vi "experiment control.vi"() -> ()   [LabVIEW 2012] (continued)
                    n363 = Greater Or Equal?(x=w828, y=w827) -> (x >= y?=w826:bool)
                    n364 = Greater?(x=w827, y=w829) -> (0:w825:bool)
                    n365 = And(x=w826, y=w825) -> (x .and. y?=w823:bool)
                  }
                  frame "TiSapph" {
                    n366 = local read "TiSapph"() -> (w833:T18)
                    n367 = Unbundle By Name(w833) -> ("scan start"=w840:dbl, "setpoint"=w836:dbl, "scan end"=w839:dbl)
                    n368 = Max & Min(x=w840, y=w839) -> (max(x,y)=w837:dbl, min(x,y)=w838:dbl)
                    n369 = Greater Or Equal?(x=w837, y=w836) -> (x >= y?=w835:bool)
                    n370 = Greater?(x=w836, y=w838) -> (0:w834:bool)
                    n371 = And(x=w835, y=w834) -> (x .and. y?=w832:bool)
                  }
                  frame "Scan" {
                    n372 = case shown="\"\"" w841 {
                      tunnel: [w849 w850] -> w842
                      tunnel: w841 -> [w843 _]
                      frame Default {
                        n373 = local read "Scan References"() -> (w848:T33)
                        n374 = Decimal String To Number(string=w843) -> (number=w847:i32)  [unwired: 2 in, 1 out]
                        n375 = Index Array(array=w848, index=w847) -> (element=w846:T57)
                        n376 = Unbundle By Name(w846) -> ("progress"=w845:u8)
                        n377 = Less?(x=w845, y=u8 100) -> (x < y?=w849:bool)
                      }
                      frame "" {
                        n378 = local read "Scan References"() -> (w852:T33)
                        n379 = for {
                          tunnel: w852 -> [w858] mode=indexing
                          tunnel: [w854] -> w851 mode=indexing
                          n380 = Unbundle By Name(w858) -> ("scan"=w853:bool, "progress"=w857:u8)
                          n381 = Less?(x=w857, y=u8 100) -> (x < y?=w855:bool)
                          n382 = And(x=w853, y=w855) -> (x .and. y?=w854:bool)
                        }
                        n383 = Or Array Elements(Boolean array=w851) -> (logical OR=w850:bool)
                      }
                    }
                  }
                  frame "Switch" {
                    n384 = local read "Slide"() -> (w859:u8)
                    n385 = Less?(x=w859, y=u8 100) -> (x < y?=w861:bool)
                  }
                }
                n386 = case shown="True" w783 {
                  tunnel: w781 -> [_ w794]
                  tunnel: w785 -> [_ w793]
                  tunnel: [w791 w792] -> w784
                  tunnel: w782 -> [w791 _]
                  frame False {
                  }
                  frame True {
                    n387 = Build Array (concatenate)(w793, w794) -> (w792:string[])
                  }
                }
              }
            }
            n388 = Reverse 1D Array(array=w765) -> (reversed array=w768:string[])
            n389 = for {
              tunnel: w769 -> [w777]
              tunnel: w768 -> [w774] mode=indexing
              shift-right: [w775] -> w766
              shift-left: w767 -> [w776]
              n390 = Enqueue Element At Opposite End(queue=w777, element=w774, error in (no error)=w776) -> (error out=w775:errorcluster)  [unwired: 1 in, 2 out]
            }
          }
          frame "Count Ions" {
            # "This command calls the custom functions specified in the programming tab"
            n391 = Index Array(array=w883) -> (element=w882:string)  [unwired: 1 in]
            n392 = Unbundle By Name(w919) -> ("TDS5034B Data"=w915:cluster{"Y":dbl[], "t0":dbl, "dt":dbl}[])
            n393 = Decimal String To Number(string=w882) -> (number=w916:i32)  [unwired: 2 in, 1 out]
            n394 = Unbundle By Name("Count Ions") -> ("Hf  time threshold"=w900:dbl, "Ion Calibration"=w901:dbl, "Hf integrated history"=w898:dbl[], "HfF history"=w897:dbl[], "History"=w886:u32, "Clear History"=w887:bool)
            n395 = Index Array(array=w915, index=w916) -> (element=w917:cluster{"Y":dbl[], "t0":dbl, "dt":dbl})
            n396 = Unbundle By Name(w917) -> ("Y"=w910:dbl[], "dt"=w902:dbl)
            n397 = Select(t=u32 1, s=w887, f=w886) -> (s? t:f=w885:u32)
            n398 = Array Subset(array=w910, length=500) -> (w913:dbl[])  [unwired: 1 in]
            n399 = call-poly <vilib>:"Mean.vi"("X"=w913) -> ("mean"=w911:dbl)  [unwired: 1 out]
            n400 = Subtract(x=w910, y=w911) -> (x-y=w909:dbl[])
            n401 = Divide(x=w900, y=w902) -> (x/y=w912:dbl)
            n402 = Split 1D Array(array=w909, index=w912) -> (first subarray=w908:dbl[], second subarray=w907:dbl[])
            n403 = Add Array Elements(numeric array=w908) -> (sum=w903:dbl)
            n404 = Add Array Elements(numeric array=w907) -> (sum=w904:dbl)
            n405 = Multiply(x=w902, y=w903) -> (x*y=w906:dbl)
            n406 = Multiply(x=w902, y=w904) -> (x*y=w905:dbl)
            n407 = Divide(x=w906, y=w901) -> (x/y=w896:dbl)
            n408 = Divide(x=w905, y=w901) -> (x/y=w895:dbl)
            n409 = Build Array (concatenate)(w896, w898) -> (w893:dbl[])
            n410 = Build Array (concatenate)(w895, w897) -> (w892:dbl[])
            n411 = Array Subset(array=w893, length=w885) -> (w889:dbl[])  [unwired: 1 in]
            n412 = Array Subset(array=w892, length=w885) -> (w888:dbl[])  [unwired: 1 in]
            n413 = call-poly <vilib>:"Mean.vi"("X"=w889) -> ("mean"=w890:dbl)  [unwired: 1 out]
            n414 = call-poly <vilib>:"Mean.vi"("X"=w888) -> ("mean"=w891:dbl)  [unwired: 1 out]
            n415 = Bundle By Name(cluster="Count Ions", "Hf integrated"=w896, "HfF"=w895, "Hf integrated history"=w889, "HfF history"=w888, "<Hf integrated>"=w890, "<HfF>"=w891) -> (w894:T34)
            n416 = local write "Count Ions"(w894) -> ()
          }
          frame "uBinary: Save" {
            # "Saves a uBinary file or loads a uBinary file."
            n417 = flat-sequence {
              tunnel: [w933] -> w923
              tunnel: w927 -> [w933]
              tunnel: w921 -> [w928]
              frame #0 {
                n418 = Unbundle By Name(w928) -> ("TDS5034B Data"=→"TDS5034B Data":cluster{"Y":dbl[], "t0":dbl, "dt":dbl}[])
                n419 = Get Date/Time String(want seconds? (F)=TRUE) -> (date string=w931:string, time string=w932:string)  [unwired: 2 in]
                n420 = local write "Time"(w932) -> ()
                n421 = local write "Date"(w931) -> ()
              }
            }
            n422 = case shown="\"Scan\"" w925 {
              selector: w925 -> [_ _ w1085 _]
              tunnel: w923 -> [w940 w960 w1086 w1092]
              tunnel: [w936 w963 w1089 w1091] -> w926
              tunnel: [w934 w962 w1088 w1096] -> w924
              tunnel: w921 -> [w934 w962 w1088 w1097]
              frame "Prompt" {
                n423 = Format Date/Time String(time format string (%c)="%Y") -> (date/time string=w943:string)  [unwired: 2 in]
                n424 = Format Date/Time String(time format string (%c)="\\%y%m%d\\") -> (date/time string=w941:string)  [unwired: 2 in]
                n425 = Concatenate Strings("X:\\" ("string"), w943, w941) -> (w946:string)
                n426 = String To Path(string=w946) -> (path=w949:path)
                n427 = call "File Dialog3"("start path"=w949, "prompt"="Save Experiment (*.ubin)", "button label"="Save", "error in"=w940, "pattern (all files)"="*.ubin") -> ("selected path"=w938:path, "error out"=w939:errorcluster)  [unwired: 7 in, 2 out]
                n428 = control-ref of="This VI"() -> (w937:refnum<vi>)
                n429 = call "ubinary_save.vi"("error in"=w939, "file (use dialog)"=w938, "VI"=w937) -> ("error out"=w936:errorcluster)  [unwired: 8 in]
              }
              frame "" {
                n430 = local read "Working Directory"() -> (w952:path)
                n431 = List Folder(path=w952, error in=w960) -> (filenames=w951:string[], error out=w959:errorcluster)  [unwired: 2 in, 2 out]
                n432 = Path To String(path=w952) -> (string=w954:string)
                n433 = Array Size(array=w951) -> (size(s)=w950:i32)
                n434 = case shown="Default" w950 {
                  tunnel: w951 -> [_ w969]
                  tunnel: [1 w966] -> w958
                  frame 0 {
                  }
                  frame Default {
                    n435 = for {
                      tunnel: w969 -> [w973] mode=indexing
                      tunnel: [w971] -> w968 mode=indexing
                      n436 = xnode "Match Regular Expression"("input string"=w973, "regular expression"="\\d+") -> ("whole match"=w972:string)  [unwired: 4 in, 4 out]
                      n437 = Decimal String To Number(string=w972) -> (number=w971:i32)  [unwired: 2 in, 1 out]
                    }
                    n438 = Array Max & Min(array=w968) -> (max value=w967:i32)  [unwired: 3 out]
                    n439 = Increment(x=w967) -> (x+1=w966:i32)
                  }
                }
                n440 = Number To Decimal String(number=w958) -> (decimal integer string=w957:string)  [unwired: 1 in]
                n441 = Concatenate Strings(w954, "\\s" ("string"), w957, ".ubin" ("string")) -> (w955:string)
                n442 = control-ref of="This VI"() -> (w964:refnum<vi>)
                n443 = String To Path(string=w955) -> (path=w961:path)
                n444 = call "ubinary_save.vi"("error in"=w959, "file (use dialog)"=w961, "VI"=w964) -> ("error out"=w963:errorcluster)  [unwired: 8 in]
              }
              frame Default {
                n445 = control-ref of="This VI"() -> (w1090:refnum<vi>)
                n446 = String To Path(string=w1085) -> (path=w1087:path)
                n447 = call "ubinary_save.vi"("error in"=w1086, "file (use dialog)"=w1087, "VI"=w1090) -> ("error out"=w1089:errorcluster)  [unwired: 8 in]
              }
              frame "Scan" {
                w1105 = "." ("substring (\"\")")
                n448 = Unbundle By Name(w1097) -> ("Scan Index"=w1098:u32, "Scan Prefix"=w1099:path, "Scan Index"=w1095:u32)
                n449 = Number To Decimal String(number=w1095) -> (decimal integer string=w1103:string)  [unwired: 1 in]
                n450 = Strip Path(path=w1099) -> (stripped path=w1101:path, name=w1106:string)
                n451 = Concatenate Strings(w1103, w1105) -> (w1104:string)
                n452 = Increment(x=w1098) -> (x+1=w1100:u32)
                n453 = Search and Replace String(input string=w1106, search string=w1105, replace string=w1104) -> (result string=w1102:string)  [unwired: 5 in, 3 out]
                n454 = Bundle By Name(cluster=w1097, "Scan Index"=w1100) -> (w1096:T52)
                n455 = Build Path(base path=w1101, name or relative path=w1102) -> (appended path=w1093:path)
                n456 = control-ref of="This VI"() -> (w1094:refnum<vi>)
                n457 = call "ubinary_save.vi"("error in"=w1092, "file (use dialog)"=w1093, "VI"=w1094) -> ("error out"=w1091:errorcluster)  [unwired: 8 in]
              }
            }
          }
          frame "uBinary: Load" {
            # "Saves a uBinary file or loads a uBinary file."
            n458 = Index Array(array=w1108, index=0) -> (element=w1107:string)
            n459 = Index Array(array=w1108, index=1) -> (element=w1111:string)
            n460 = case shown="\"False\", Default" w1111 {
              selector: w1111 -> [w1119 _]
              tunnel: w1115 -> [w1121 w1134]
              tunnel: [w1121 w1124] -> w1114
              tunnel: [w1120 w1123] -> w1113
              frame "False", Default {
                n461 = String To Path(string=w1119) -> (path=w1120:path)
              }
              frame "" {
                n462 = Format Date/Time String(time format string (%c)="%Y") -> (date/time string=w1127:string)  [unwired: 2 in]
                n463 = Format Date/Time String(time format string (%c)="\\%y%m%d\\") -> (date/time string=w1125:string)  [unwired: 2 in]
                n464 = Concatenate Strings("X:\\" ("string"), w1127, w1125) -> (w1130:string)
                n465 = String To Path(string=w1130) -> (path=w1133:path)
                n466 = call "File Dialog2"("start path"=w1133, "prompt"="Load Experiment (*.ubin)", "button label"="Load", "error in"=w1134, "pattern (all files)"="*.ubin") -> ("selected path"=w1123:path, "error out"=w1124:errorcluster)  [unwired: 7 in, 2 out]
              }
            }
            n467 = control-ref of="This VI"() -> (w1112:refnum<vi>)
            n468 = call "ubinary_load.vi"("error in"=w1114, "control"=w1107, "file (use dialog)"=w1113, "VI"=w1112) -> ("error out"=w1118:errorcluster)  [unwired: 7 in]
          }
          frame "uBinary2" {
            # "First, modify Save"
            # "Saves a uBinary file or loads a uBinary file."
            n469 = Match Pattern(string=w1144, regular expression=",") -> (before substring=w1138:string, after substring=w1136:string, offset past match=w1137:i32)  [unwired: 1 in, 1 out]
            n470 = case shown="\"Load\"" w1138 {
              tunnel: [w1153 w1400 w1421] -> w1142
              tunnel: w1143 -> [w1145 w1399 w1423]
              tunnel: w1140 -> [w1146 _ w1419]
              tunnel: [w1149 w1402 w1418] -> w1141
              tunnel: w1140 -> [w1149 w1401 w1417]
              tunnel: w1137 -> [w1148 _ _]
              tunnel: w1136 -> [w1147 _ _]
              tunnel: w1135 -> [_ w1394 w1413]
              frame "Save", Default {
                n471 = case shown="0, Default" w1148 {
                  tunnel: w1145 -> [w1156 w1161]
                  tunnel: [w1156 w1160] -> w1152
                  tunnel: [w1154 w1159] -> w1151
                  tunnel: [FALSE ("cancelled") w1158] -> w1150
                  tunnel: w1147 -> [w1155 _]
                  frame 0, Default {
                    n472 = String To Path(string=w1155) -> (path=w1154:path)
                  }
                  frame -1 {
                    n473 = Format Date/Time String(time format string (%c)="%Y") -> (date/time string=w1164:string)  [unwired: 2 in]
                    n474 = Format Date/Time String(time format string (%c)="\\%y%m%d\\") -> (date/time string=w1162:string)  [unwired: 2 in]
                    n475 = Concatenate Strings("X:\\" ("string"), w1164, w1162) -> (w1167:string)
                    n476 = String To Path(string=w1167) -> (path=w1170:path)
                    n477 = call "File Dialog4"("start path"=w1170, "prompt"="Save Experiment (*.ubin)", "button label"="Save", "error in"=w1161) -> ("selected path"=w1159:path, "cancelled"=w1158:bool, "error out"=w1160:errorcluster)  [unwired: 8 in, 1 out]
                  }
                }
                n478 = case shown="False" w1150 {
                  tunnel: [w1174 w1393] -> w1153
                  tunnel: w1152 -> [w1173 w1393]
                  tunnel: w1151 -> [w1172 _]
                  tunnel: w1146 -> [w1171 _]
                  frame False {
                    # "Then add a case to handle the tag"
                    # "Add your tag to the list"
                    n479 = call "begin_ubin.vi"("error in"=w1173, "file"=w1172) -> ("error out"=w1178:errorcluster, "refnum out"=w1179:refnum<file>)  [unwired: 8 in]
                    n480 = for {
                      tunnel: string[] ["Time", "DIO64", "DAC", "Scan", "Lasers", "AOM DDS", "Trap DDS", "Commands", "Wavemaster", "Frequency", "Microwave", "Measurements", "Switches", "Data", "Trap"] -> [w1181] mode=indexing
                      shift-right: [w1183] -> w1177
                      shift-left: w1179 -> [w1185]
                      shift-right: [w1182] -> w1176
                      shift-left: w1178 -> [w1184]
                      tunnel: w1171 -> [w1180]
                      n481 = case shown="\"Wavemaster\"" w1181 {
                        selector: w1181 -> [_ w1199 w1213 w1226 w1243 w1255 w1267 w1282 w1296 w1309 w1321 w1333 w1347 w1359 w1375 w1387]
                        tunnel: w1185 -> [w1187 w1204 w1218 w1231 w1248 w1260 w1272 w1287 w1301 w1314 w1326 w1338 w1352 w1364 w1380 w1392]
                        tunnel: w1184 -> [w1186 w1195 w1206 w1220 w1234 w1250 w1262 w1274 w1292 w1303 w1316 w1328 w1342 w1354 w1366 w1383]
                        tunnel: [w1187 w1203 w1217 w1230 w1247 w1259 w1271 w1286 w1300 w1313 w1325 w1337 w1351 w1363 w1379 w1391] -> w1183
                        tunnel: [w1186 w1202 w1216 w1229 w1246 w1258 w1270 w1285 w1299 w1312 w1324 w1336 w1350 w1362 w1378 w1390] -> w1182
                        tunnel: w1180 -> [_ _ _ _ _ _ _ _ _ _ _ _ _ _ w1370 _]
                        frame "False", Default {
                        }
                        frame "DIO64" {
                          n482 = local read "Frames and Rep Rate"() -> (w1189:cluster{"Frames":i32, "Repetition Rate":dbl})
                          n483 = local read "Channel Labels"() -> (w1191:T10)
                          n484 = local read "Current Chops"() -> (w1190:u16[])
                          n485 = local read "Chop Labels"() -> (w1188:string[])
                          n486 = local read "DIO64 Tasks"() -> (w1192:T4)
                          n487 = local read "DIO64"() -> (w1193:T3)
                          n488 = Bundle("DIO64"=w1193, "DIO64 Tasks"=w1192, "Channel Labels"=w1191, "Current Chops"=w1190, "Frames and Rep Rate"=w1189, "Chop Labels"=w1188) -> (w1196:T58)  [unwired: 1 in]
                          n489 = call "ubinary.vi"("Cluster"=w1196) -> ("Header"=w1198:cluster{"Element Names":string[], u8[]})  [unwired: 9 in, 1 out]
                          n490 = Bundle("Header"=w1198, w1196) -> (w1197:T59)  [unwired: 1 in]
                          n491 = call "save_ubin_tag.vi"("error in"=w1195, "Name"=w1199, "refnum"=w1204) -> ("error out"=w1194:errorcluster, "refnum out"=w1201:refnum<file>)  [unwired: 7 in]
                          n492 = Write to Binary File(file (use dialog)=w1201, data=w1197, error in=w1194, 9:T45."native, host order" ("byte order (0:big-endian, network order)")) -> (refnum out=w1203:refnum<file>, error out=w1202:errorcluster)  [unwired: 2 in, 1 out]
                        }
                        frame "DAC" {
                          n493 = local read "DAC Schedule"() -> (w1210:T6)
                          n494 = local read "DAC Kick 2"() -> (w1208:T8)
                          n495 = local read "DAC Tasks"() -> (w1209:T8)
                          n496 = Bundle("DAC Schedule"=w1210, "DAC Tasks"=w1209, "DAC Kick 2"=w1208) -> (w1207:T60)  [unwired: 1 in]
                          n497 = call "ubinary.vi"("Cluster"=w1207) -> ("Header"=w1212:cluster{"Element Names":string[], u8[]})  [unwired: 9 in, 1 out]
                          n498 = Bundle("Header"=w1212, w1207) -> (w1211:T61)  [unwired: 1 in]
                          n499 = call "save_ubin_tag.vi"("error in"=w1206, "Name"=w1213, "refnum"=w1218) -> ("error out"=w1205:errorcluster, "refnum out"=w1215:refnum<file>)  [unwired: 7 in]
                          n500 = Write to Binary File(file (use dialog)=w1215, data=w1211, error in=w1205, 9:T45."native, host order" ("byte order (0:big-endian, network order)")) -> (refnum out=w1217:refnum<file>, error out=w1216:errorcluster)  [unwired: 2 in, 1 out]
                        }
                        frame "Scan" {
                          n501 = local read "Scan References"() -> (w1223:T33)
                          n502 = local read "Scan Variables"() -> (w1222:T32)
                          n503 = Bundle("Scan References"=w1223, "Scan Variables"=w1222) -> (w1221:T62)  [unwired: 1 in]
                          n504 = call "ubinary.vi"("Cluster"=w1221) -> ("Header"=w1225:cluster{"Element Names":string[], u8[]})  [unwired: 9 in, 1 out]
                          n505 = Bundle("Header"=w1225, w1221) -> (w1224:T63)  [unwired: 1 in]
                          n506 = call "save_ubin_tag.vi"("error in"=w1220, "Name"=w1226, "refnum"=w1231) -> ("error out"=w1219:errorcluster, "refnum out"=w1228:refnum<file>)  [unwired: 7 in]
                          n507 = Write to Binary File(file (use dialog)=w1228, data=w1224, error in=w1219, 9:T45."native, host order" ("byte order (0:big-endian, network order)")) -> (refnum out=w1230:refnum<file>, error out=w1229:errorcluster)  [unwired: 2 in, 1 out]
                        }
                        frame "Lasers" {
                          n508 = local read "TiSapph"() -> (w1232:T18)
                          n509 = local read "Toptica"() -> (w1236:T19)
                          n510 = local read "Jessica"() -> (w1240:T17)
                          n511 = local read "Bertha"() -> (w1239:T22)
                          n512 = local read "Stella"() -> (w1237:T20)
                          n513 = local read "Cora"() -> (w1238:T21)
                          n514 = Bundle("Jessica"=w1240, "Bertha"=w1239, "Cora"=w1238, "Stella"=w1237, "Toptica"=w1236, "TiSapph"=w1232) -> (w1235:T64)  [unwired: 1 in]
                          n515 = call "ubinary.vi"("Cluster"=w1235) -> ("Header"=w1242:cluster{"Element Names":string[], u8[]})  [unwired: 9 in, 1 out]
                          n516 = Bundle("Header"=w1242, w1235) -> (w1241:T65)  [unwired: 1 in]
                          n517 = call "save_ubin_tag.vi"("error in"=w1234, "Name"=w1243, "refnum"=w1248) -> ("error out"=w1233:errorcluster, "refnum out"=w1245:refnum<file>)  [unwired: 7 in]
                          n518 = Write to Binary File(file (use dialog)=w1245, data=w1241, error in=w1233, 9:T45."native, host order" ("byte order (0:big-endian, network order)")) -> (refnum out=w1247:refnum<file>, error out=w1246:errorcluster)  [unwired: 2 in, 1 out]
                        }
                        frame "AOM DDS" {
                          n519 = local read "DDS"() -> (w1252:T25)
                          n520 = Bundle("DDS"=w1252) -> (w1251:T66)  [unwired: 1 in]
                          n521 = call "ubinary.vi"("Cluster"=w1251) -> ("Header"=w1254:cluster{"Element Names":string[], u8[]})  [unwired: 9 in, 1 out]
                          n522 = Bundle("Header"=w1254, w1251) -> (w1253:T67)  [unwired: 1 in]
                          n523 = call "save_ubin_tag.vi"("error in"=w1250, "Name"=w1255, "refnum"=w1260) -> ("error out"=w1249:errorcluster, "refnum out"=w1257:refnum<file>)  [unwired: 7 in]
                          n524 = Write to Binary File(file (use dialog)=w1257, data=w1253, error in=w1249, 9:T45."native, host order" ("byte order (0:big-endian, network order)")) -> (refnum out=w1259:refnum<file>, error out=w1258:errorcluster)  [unwired: 2 in, 1 out]
                        }
                        frame "Trap DDS" {
                          n525 = local read "Trap DDS"() -> (w1264:T26)
                          n526 = Bundle("Trap DDS"=w1264) -> (w1263:T68)  [unwired: 1 in]
                          n527 = call "ubinary.vi"("Cluster"=w1263) -> ("Header"=w1266:cluster{"Element Names":string[], u8[]})  [unwired: 9 in, 1 out]
                          n528 = Bundle("Header"=w1266, w1263) -> (w1265:T69)  [unwired: 1 in]
                          n529 = call "save_ubin_tag.vi"("error in"=w1262, "Name"=w1267, "refnum"=w1272) -> ("error out"=w1261:errorcluster, "refnum out"=w1269:refnum<file>)  [unwired: 7 in]
                          n530 = Write to Binary File(file (use dialog)=w1269, data=w1265, error in=w1261, 9:T45."native, host order" ("byte order (0:big-endian, network order)")) -> (refnum out=w1271:refnum<file>, error out=w1270:errorcluster)  [unwired: 2 in, 1 out]
                        }
                        frame "Commands" {
                          n531 = local read "Measure Commands"() -> (w1279:string)
                          n532 = local read "Test Commands"() -> (w1278:string)
                          n533 = local read "Functions"() -> (w1277:cluster{"Name":string, "Body":string}[])
                          n534 = local read "Chops"() -> (w1273:cluster{"Chops":u16[]}[])
                          n535 = Bundle("Measure Commands"=w1279, "Test Commands"=w1278, "Functions"=w1277, "Chops"=w1273) -> (w1276:T70)  [unwired: 1 in]
                          n536 = call "ubinary.vi"("Cluster"=w1276) -> ("Header"=w1281:cluster{"Element Names":string[], u8[]})  [unwired: 9 in, 1 out]
                          n537 = Bundle("Header"=w1281, w1276) -> (w1280:T71)  [unwired: 1 in]
                          n538 = call "save_ubin_tag.vi"("error in"=w1274, "Name"=w1282, "refnum"=w1287) -> ("error out"=w1275:errorcluster, "refnum out"=w1284:refnum<file>)  [unwired: 7 in]
                          n539 = Write to Binary File(file (use dialog)=w1284, data=w1280, error in=w1275, 9:T45."native, host order" ("byte order (0:big-endian, network order)")) -> (refnum out=w1286:refnum<file>, error out=w1285:errorcluster)  [unwired: 2 in, 1 out]
                        }
                        frame "Time" {
                          n540 = Get Date/Time String(want seconds? (F)=TRUE) -> (date string=w1290:string, time string=w1289:string)  [unwired: 2 in]
                          n541 = local write "Date"(w1290) -> ()
                          n542 = local write "Time"(w1289) -> ()
                          n543 = Bundle("date string"=w1290, "time string"=w1289) -> (w1293:T72)  [unwired: 1 in]
                          n544 = call "ubinary.vi"("Cluster"=w1293) -> ("Header"=w1295:cluster{"Element Names":string[], u8[]})  [unwired: 9 in, 1 out]
                          n545 = Bundle("Header"=w1295, w1293) -> (w1294:T73)  [unwired: 1 in]
                          n546 = call "save_ubin_tag.vi"("error in"=w1292, "Name"=w1296, "refnum"=w1301) -> ("error out"=w1291:errorcluster, "refnum out"=w1298:refnum<file>)  [unwired: 7 in]
                          n547 = Write to Binary File(file (use dialog)=w1298, data=w1294, error in=w1291, 9:T45."native, host order" ("byte order (0:big-endian, network order)")) -> (refnum out=w1300:refnum<file>, error out=w1299:errorcluster)  [unwired: 2 in, 1 out]
                        }
                        frame "Switches" {
                          n548 = local read "Switch Settings"() -> (w1305:T9)
                          n549 = local read "Machine State"() -> (w1306:T1)
                          n550 = Bundle("Machine State"=w1306, "Switch Settings"=w1305) -> (w1304:T74)  [unwired: 1 in]
                          n551 = call "ubinary.vi"("Cluster"=w1304) -> ("Header"=w1308:cluster{"Element Names":string[], u8[]})  [unwired: 9 in, 1 out]
                          n552 = Bundle("Header"=w1308, w1304) -> (w1307:T75)  [unwired: 1 in]
                          n553 = call "save_ubin_tag.vi"("error in"=w1303, "Name"=w1309, "refnum"=w1314) -> ("error out"=w1302:errorcluster, "refnum out"=w1311:refnum<file>)  [unwired: 7 in]
                          n554 = Write to Binary File(file (use dialog)=w1311, data=w1307, error in=w1302, 9:T45."native, host order" ("byte order (0:big-endian, network order)")) -> (refnum out=w1313:refnum<file>, error out=w1312:errorcluster)  [unwired: 2 in, 1 out]
                        }
                        frame "Wavemaster" {
                          n555 = local read "Wavemaster"() -> (w1318:T23)
                          n556 = Bundle("Wavemaster"=w1318) -> (w1317:T76)  [unwired: 1 in]
                          n557 = call "ubinary.vi"("Cluster"=w1317) -> ("Header"=w1320:cluster{"Element Names":string[], u8[]})  [unwired: 9 in, 1 out]
                          n558 = Bundle("Header"=w1320, w1317) -> (w1319:T77)  [unwired: 1 in]
                          n559 = call "save_ubin_tag.vi"("error in"=w1316, "Name"=w1321, "refnum"=w1326) -> ("error out"=w1315:errorcluster, "refnum out"=w1323:refnum<file>)  [unwired: 7 in]
                          n560 = Write to Binary File(file (use dialog)=w1323, data=w1319, error in=w1315, 9:T45."native, host order" ("byte order (0:big-endian, network order)")) -> (refnum out=w1325:refnum<file>, error out=w1324:errorcluster)  [unwired: 2 in, 1 out]
                        }
                        frame "Microwave" {
                          n561 = local read "HP8341B"() -> (w1330:T27)
                          n562 = Bundle("HP8341B"=w1330) -> (w1329:T78)  [unwired: 1 in]
                          n563 = call "ubinary.vi"("Cluster"=w1329) -> ("Header"=w1332:cluster{"Element Names":string[], u8[]})  [unwired: 9 in, 1 out]
                          n564 = Bundle("Header"=w1332, w1329) -> (w1331:T79)  [unwired: 1 in]
                          n565 = call "save_ubin_tag.vi"("error in"=w1328, "Name"=w1333, "refnum"=w1338) -> ("error out"=w1327:errorcluster, "refnum out"=w1335:refnum<file>)  [unwired: 7 in]
                          n566 = Write to Binary File(file (use dialog)=w1335, data=w1331, error in=w1327, 9:T45."native, host order" ("byte order (0:big-endian, network order)")) -> (refnum out=w1337:refnum<file>, error out=w1336:errorcluster)  [unwired: 2 in, 1 out]
                        }
                        frame "Measurements" {
                          n567 = local read "Temperature Monitor"() -> (w1339:T29)
                          n568 = local read "Magnetometer"() -> (w1340:T28)
                          n569 = local read "QuadDVM"() -> (w1344:T31)
                          n570 = Bundle("QuadDVM"=w1344, "Magnetometer"=w1340, "Temperature Monitor"=w1339) -> (w1343:T80)  [unwired: 1 in]
                          n571 = call "ubinary.vi"("Cluster"=w1343) -> ("Header"=w1346:cluster{"Element Names":string[], u8[]})  [unwired: 9 in, 1 out]
                          n572 = Bundle("Header"=w1346, w1343) -> (w1345:T81)  [unwired: 1 in]
                          n573 = call "save_ubin_tag.vi"("error in"=w1342, "Name"=w1347, "refnum"=w1352) -> ("error out"=w1341:errorcluster, "refnum out"=w1349:refnum<file>)  [unwired: 7 in]
                          n574 = Write to Binary File(file (use dialog)=w1349, data=w1345, error in=w1341, 9:T45."native, host order" ("byte order (0:big-endian, network order)")) -> (refnum out=w1351:refnum<file>, error out=w1350:errorcluster)  [unwired: 2 in, 1 out]
                        }
                        frame "Frequency" {
                          n575 = local read "Frequency Counter"() -> (w1356:T30)
                          n576 = Bundle("Frequency Counter"=w1356) -> (w1355:T82)  [unwired: 1 in]
                          n577 = call "ubinary.vi"("Cluster"=w1355) -> ("Header"=w1358:cluster{"Element Names":string[], u8[]})  [unwired: 9 in, 1 out]
                          n578 = Bundle("Header"=w1358, w1355) -> (w1357:T83)  [unwired: 1 in]
                          n579 = call "save_ubin_tag.vi"("error in"=w1354, "Name"=w1359, "refnum"=w1364) -> ("error out"=w1353:errorcluster, "refnum out"=w1361:refnum<file>)  [unwired: 7 in]
                          n580 = Write to Binary File(file (use dialog)=w1361, data=w1357, error in=w1353, 9:T45."native, host order" ("byte order (0:big-endian, network order)")) -> (refnum out=w1363:refnum<file>, error out=w1362:errorcluster)  [unwired: 2 in, 1 out]
                        }
                        frame "Data" {
                          n581 = local read "TDS5034B Oscilloscope"() -> (w1372:T24)
                          n582 = local read "TDS2014 Oscilloscope"() -> (w1371:T24)
                          n583 = Unbundle By Name(w1370) -> ("TDS5034B Data"=w1369:cluster{"Y":dbl[], "t0":dbl, "dt":dbl}[], "TDS2014 Data"=w1368:cluster{"Y":dbl[], "t0":dbl, "dt":dbl}[])
                          n584 = Bundle("TDS5034B Oscilloscope"=w1372, "TDS2014 Oscilloscope"=w1371, "TDS5034B Data"=w1369, "TDS2014 Data"=w1368) -> (w1367:T84)  [unwired: 1 in]
                          n585 = call "ubinary.vi"("Cluster"=w1367) -> ("Header"=w1374:cluster{"Element Names":string[], u8[]})  [unwired: 9 in, 1 out]
                          n586 = Bundle("Header"=w1374, w1367) -> (w1373:T85)  [unwired: 1 in]
                          n587 = call "save_ubin_tag.vi"("error in"=w1366, "Name"=w1375, "refnum"=w1380) -> ("error out"=w1365:errorcluster, "refnum out"=w1377:refnum<file>)  [unwired: 7 in]
                          n588 = Write to Binary File(file (use dialog)=w1377, data=w1373, error in=w1365, 9:T45."native, host order" ("byte order (0:big-endian, network order)")) -> (refnum out=w1379:refnum<file>, error out=w1378:errorcluster)  [unwired: 2 in, 1 out]
                        }
                        frame "Trap" {
                          n589 = local read "Trap Agilent"() -> (w1381:T13)
                          n590 = Bundle("Trap Agilent"=w1381) -> (w1384:T86)  [unwired: 1 in]
                          n591 = call "ubinary.vi"("Cluster"=w1384) -> ("Header"=w1386:cluster{"Element Names":string[], u8[]})  [unwired: 9 in, 1 out]
                          n592 = Bundle("Header"=w1386, w1384) -> (w1385:T87)  [unwired: 1 in]
                          n593 = call "save_ubin_tag.vi"("error in"=w1383, "Name"=w1387, "refnum"=w1392) -> ("error out"=w1382:errorcluster, "refnum out"=w1389:refnum<file>)  [unwired: 7 in]
                          n594 = Write to Binary File(file (use dialog)=w1389, data=w1385, error in=w1382, 9:T45."native, host order" ("byte order (0:big-endian, network order)")) -> (refnum out=w1391:refnum<file>, error out=w1390:errorcluster)  [unwired: 2 in, 1 out]
                        }
                      }
                    }
                    n595 = Close File(refnum=w1177, error in=w1176) -> (error out=w1174:errorcluster)  [unwired: 1 out]
                  }
                  frame True {
                  }
                }
              }
              frame "Save Scan" {
                w1411 = "." ("substring (\"\")")
                n596 = Unbundle By Name(w1401) -> ("Scan Index"=w1404:u32, "Scan Prefix"=w1405:path, "Scan Index"=w1403:u32)
                n597 = Number To Decimal String(number=w1403) -> (decimal integer string=w1409:string)  [unwired: 1 in]
                n598 = Increment(x=w1404) -> (x+1=w1406:u32)
                n599 = Strip Path(path=w1405) -> (stripped path=w1407:path, name=w1412:string)
                n600 = Concatenate Strings(w1409, w1411) -> (w1410:string)
                n601 = Bundle By Name(cluster=w1401, "Scan Index"=w1406) -> (w1402:T52)
                n602 = Search and Replace String(input string=w1412, search string=w1411, replace string=w1410, error in=w1399) -> (result string=w1408:string, error out=w1400:errorcluster)  [unwired: 4 in, 2 out]
                n603 = Build Path(base path=w1407, name or relative path=w1408) -> (appended path=w1398:path)
                n604 = Path To String(path=w1398) -> (string=w1396:string)
                n605 = Concatenate Strings("ubinary2 >> Save," ("string"), w1396) -> (w1395:string)
                n606 = Enqueue Element At Opposite End(queue=w1394, element=w1395) -> ()  [unwired: 2 in, 3 out]
              }
              frame "Load" {
                n607 = Format Date/Time String(time format string (%c)="%Y") -> (date/time string=w1426:string)  [unwired: 2 in]
                n608 = Format Date/Time String(time format string (%c)="\\%y%m%d\\") -> (date/time string=w1424:string)  [unwired: 2 in]
                n609 = Concatenate Strings("X:\\" ("string"), w1426, w1424) -> (w1429:string)
                n610 = String To Path(string=w1429) -> (path=w1432:path)
                n611 = call "File Dialog5"("start path"=w1432, "prompt"="Load Experiment (*.ubin)", "button label"="Load", "error in"=w1423) -> ("selected path"=w1420:path, "exists"=w1434:bool, "cancelled"=w1433:bool, "error out"=w1416:errorcluster)  [unwired: 8 in]
                n612 = Not(x=w1433) -> (.not. x?=w1435:bool)
                n613 = call "load_select.vi"("error in"=w1416) -> ("error out"=w1415:errorcluster, "Array"=w1414:string[])  [unwired: 9 in]
                n614 = And(x=w1435, y=w1434) -> (x .and. y?=w1422:bool)
                n615 = case shown="True" w1422 {
                  tunnel: w1415 -> [w1439 w1445]
                  tunnel: [w1439 w1449] -> w1421
                  tunnel: w1420 -> [_ w1448]
                  tunnel: w1419 -> [_ w1444]
                  tunnel: [w1438 w1443] -> w1418
                  tunnel: w1417 -> [w1438 w1442]
                  tunnel: w1414 -> [_ w1441]
                  tunnel: w1413 -> [w1436 w1440]
                  frame False {
                    n616 = Enqueue Element At Opposite End(queue=w1436, element="Debug: Console >> Load cancelled or file does not exist!") -> ()  [unwired: 2 in, 3 out]
                  }
                  frame True {
                    n617 = Open/Create/Replace File(file path (use dialog)=w1448, error in=w1445) -> (refnum out=w1447:refnum<file>, error out=w1446:errorcluster)  [unwired: 4 in, 1 out]
                    n618 = for {
                      tunnel: w1441 -> [w1456] mode=indexing
                      shift-right: [w1458] -> w1450
                      shift-left: w1447 -> [w1460]
                      shift-right: [w1457] -> w1451
                      shift-left: w1446 -> [w1459]
                      tunnel: w1444 -> [w1455]
                      tunnel: [w1454] -> w1443
                      tunnel: w1442 -> [w1453]
                      tunnel: w1440 -> [w1452]
                      n619 = case shown="\"Wavemaster\"" w1456 {
                        selector: w1456 -> [_ w1480 w1509 w1534 w1563 w1588 w1609 w1630 w1651 w1672 w1696 w1721 w1744 w1771]
                        tunnel: w1460 -> [w1463 w1478 w1507 w1532 w1561 w1586 w1607 w1628 w1649 w1670 w1694 w1719 w1742 w1769]
                        tunnel: w1459 -> [w1462 w1479 w1508 w1533 w1562 w1587 w1608 w1629 w1650 w1671 w1695 w1720 w1743 w1770]
                        tunnel: [w1463 w1473 w1502 w1527 w1556 w1581 w1602 w1623 w1644 w1665 w1689 w1714 w1737 w1764] -> w1458
                        tunnel: [w1462 w1471 w1500 w1525 w1554 w1579 w1600 w1621 w1642 w1663 w1687 w1712 w1735 w1762] -> w1457
                        tunnel: w1455 -> [_ _ _ _ _ _ _ _ _ _ _ _ _ w1756]
                        tunnel: [w1461 w1468 w1497 w1524 w1545 w1574 w1595 w1616 w1637 w1658 w1680 w1706 w1729 w1753] -> w1454
                        tunnel: w1453 -> [w1461 w1468 w1497 w1524 w1545 w1574 w1595 w1616 w1637 w1658 w1680 w1706 w1729 w1752]
                        tunnel: w1452 -> [_ w1464 w1495 w1523 w1544 w1572 w1593 w1615 w1636 w1657 w1678 w1705 w1728 w1751]
                        frame "False", Default {
                        }
                        frame "DIO64" {
                          n620 = local read "Frames and Rep Rate"() -> (w1467:cluster{"Frames":i32, "Repetition Rate":dbl})
                          n621 = call "seek_tag.vi"("error in"=w1479, "Name"=w1480, "refnum"=w1478) -> ("error out"=w1476:errorcluster, "error"=w1469:string, "refnum"=w1477:refnum<file>)  [unwired: 6 in]
                          n622 = local read "Channel Labels"() -> (w1484:T10)
                          n623 = local read "Current Chops"() -> (w1483:u16[])
                          n624 = local read "Chop Labels"() -> (w1466:string[])
                          n625 = local read "DIO64 Tasks"() -> (w1485:T4)
                          n626 = local read "DIO64"() -> (w1486:T3)
                          n627 = Concatenate Strings("Debug: Console >> " ("prompt (Open existing file)"), w1469) -> (w1465:string)
                          n628 = Bundle("DIO64"=w1486, "DIO64 Tasks"=w1485, "Channel Labels"=w1484, "Current Chops"=w1483, "Frames and Rep Rate"=w1467, "Chop Labels"=w1466) -> (w1481:T58)  [unwired: 1 in]
                          n629 = call "ubinary.vi"("Cluster"=w1481) -> ("Header"=w1482:cluster{"Element Names":string[], u8[]})  [unwired: 9 in, 1 out]
                          n630 = Bundle("Header"=w1482, w1481) -> (w1474:T59)  [unwired: 1 in]
                          n631 = Read from Binary File(5:w1474, 8:w1476, 9:T45."native, host order" ("byte order (0:big-endian, network order)"), 11:w1477) -> (0:w1471:errorcluster, 2:w1472:T59, 3:w1473:refnum<file>)  [unwired: 2 in, 1 out]
                          n632 = case shown="No Error" w1471 {
                            tunnel: w1472 -> [w1494 _]
                            frame No Error {
                              n633 = Unbundle(w1494) -> (w1493:T58)  [unwired: 1 out]
                              n634 = Unbundle By Name(w1493) -> ("DIO64"=w1488:T3, "DIO64 Tasks"=w1489:T4, "Channel Labels"=w1487:T10, "Current Chops"=w1492:u16[], "Frames and Rep Rate"=w1491:cluster{"Frames":i32, "Repetition Rate":dbl}, "Chop Labels"=w1490:string[])
                              n635 = local write "DIO64 Tasks"(w1489) -> ()
                              n636 = local write "Channel Labels"(w1487) -> ()
                              n637 = local write "Current Chops"(w1492) -> ()
                              n638 = local write "Frames and Rep Rate"(w1491) -> ()
                              n639 = local write "Chop Labels"(w1490) -> ()
                              n640 = local write "DIO64"(w1488) -> ()
                            }
                            frame Error {
                            }
                          }
                          n641 = Enqueue Element At Opposite End(queue=w1464, element=w1465) -> ()  [unwired: 2 in, 3 out]
                        }
                        frame "DAC" {
                          n642 = call "seek_tag.vi"("error in"=w1508, "Name"=w1509, "refnum"=w1507) -> ("error out"=w1505:errorcluster, "error"=w1498:string, "refnum"=w1506:refnum<file>)  [unwired: 6 in]
                          n643 = local read "DAC Schedule"() -> (w1514:T6)
                          n644 = local read "DAC Kick 2"() -> (w1512:T8)
                          n645 = local read "DAC Tasks"() -> (w1513:T8)
                          n646 = Concatenate Strings("Debug: Console >> " ("prompt (Open existing file)"), w1498) -> (w1496:string)
                          n647 = Bundle("DAC Schedule"=w1514, "DAC Tasks"=w1513, "DAC Kick 2"=w1512) -> (w1510:T60)  [unwired: 1 in]
                          n648 = call "ubinary.vi"("Cluster"=w1510) -> ("Header"=w1511:cluster{"Element Names":string[], u8[]})  [unwired: 9 in, 1 out]
                          n649 = Bundle("Header"=w1511, w1510) -> (w1503:T61)  [unwired: 1 in]
                          n650 = Read from Binary File(5:w1503, 8:w1505, 9:T45."native, host order" ("byte order (0:big-endian, network order)"), 11:w1506) -> (0:w1500:errorcluster, 2:w1501:T61, 3:w1502:refnum<file>)  [unwired: 2 in, 1 out]
                          n651 = case shown="No Error" w1500 {
                            tunnel: w1501 -> [w1519 _]
                            frame No Error {
                              n652 = Unbundle(w1519) -> (w1518:T60)  [unwired: 1 out]
                              n653 = Unbundle By Name(w1518) -> ("DAC Schedule"=w1517:T6, "DAC Tasks"=w1516:T8, "DAC Kick 2"=w1515:T8)
                              n654 = local write "DAC Schedule"(w1517) -> ()
                              n655 = local write "DAC Kick 2"(w1515) -> ()
                              n656 = local write "DAC Tasks"(w1516) -> ()
                            }
                            frame Error {
                            }
                          }
                          n657 = Enqueue Element At Opposite End(queue=w1495, element=w1496) -> ()  [unwired: 2 in, 3 out]
                        }
                        frame "Scan" {
                          n658 = local read "Scan Variables"() -> (w1537:T32)
                          n659 = local read "Scan References"() -> (w1538:T33)
                          n660 = call "seek_tag.vi"("error in"=w1533, "Name"=w1534, "refnum"=w1532) -> ("error out"=w1530:errorcluster, "error"=w1522:string, "refnum"=w1531:refnum<file>)  [unwired: 6 in]
                          n661 = Concatenate Strings("Debug: Console >> " ("prompt (Open existing file)"), w1522) -> (w1521:string)
                          n662 = Bundle("Scan References"=w1538, "Scan Variables"=w1537) -> (w1535:T62)  [unwired: 1 in]
                          n663 = call "ubinary.vi"("Cluster"=w1535) -> ("Header"=w1536:cluster{"Element Names":string[], u8[]})  [unwired: 9 in, 1 out]
                          n664 = Bundle("Header"=w1536, w1535) -> (w1528:T63)  [unwired: 1 in]
                          n665 = Read from Binary File(5:w1528, 8:w1530, 9:T45."native, host order" ("byte order (0:big-endian, network order)"), 11:w1531) -> (0:w1525:errorcluster, 2:w1526:T63, 3:w1527:refnum<file>)  [unwired: 2 in, 1 out]
                          n666 = case shown="No Error" w1525 {
                            tunnel: w1526 -> [w1542 _]
                            frame No Error {
                              n667 = Unbundle(w1542) -> (w1541:T62)  [unwired: 1 out]
                              n668 = Unbundle By Name(w1541) -> ("Scan References"=w1540:T33, "Scan Variables"=w1539:T32)
                              n669 = local write "Scan Variables"(w1539) -> ()
                              n670 = local write "Scan References"(w1540) -> ()
                            }
                            frame Error {
                            }
                          }
